vi "4461 Replace AO Ch.vi"(8 "error in (no error)":errorcluster, 10 "Lockin.DAQ (NEW)":refnum<class "Lockin.DAQ.lvclass">, 11 "Lockin.DAQ (OLD)":refnum<class "Lockin.DAQ.lvclass">) -> (0 "error out":errorcluster, 3 "Lockin.DAQ out":refnum<class "Lockin.DAQ.lvclass">)   [LabVIEW 2016, in "Lockin.DAQ.lvclass"]
uses:
  Lockin.DAQ.lvclass
  Lockin.DAQ.lvclass/Lockin.DAQ.ctl
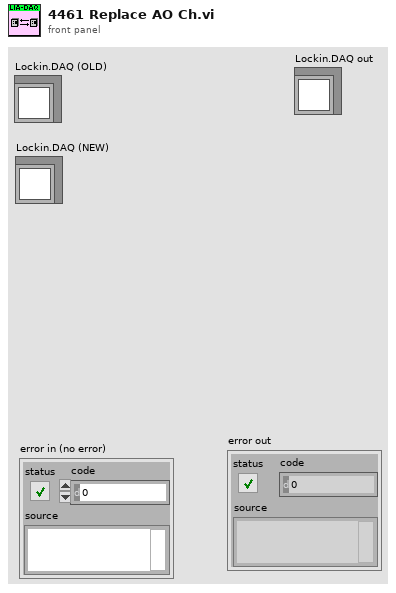
[diagram p1: front panel]
types:
  T1 = typedef "Lockin.DAQ.lvclass/AO-cluster.ctl" = cluster{"Ch":i32[], "Amp (V)":dbl[], "DC (V)":dbl[], "f (Hz)":dbl[], "Phase (°)":dbl[], "Function":T2[], "Sweep?":bool[]}
  T2 = typedef "Lockin.DAQ.lvclass/Function-enum.ctl" = enum16{"Sine", "Triangle", "Square", "Sawtooth"}
  T3 = typedef "Lockin.DAQ.lvclass/REF-cluster.ctl" = cluster{"Ch":i32[], " f (Hz)":dbl[], "Phase (°)":dbl[], "TC (s)":dbl[], "order":i32[]}
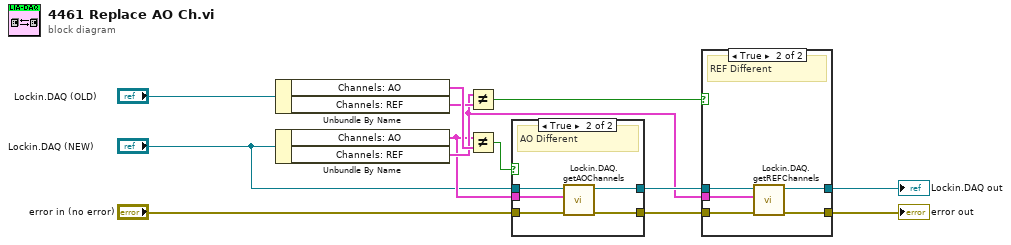
[diagram p0: block diagram]
diagram:
  n1 = Unbundle By Name("Lockin.DAQ (OLD)") -> ("Channels: AO"=w12:T1, "Channels: REF"=w11:T3)
  n2 = Unbundle By Name("Lockin.DAQ (NEW)") -> ("Channels: AO"=w2:T1, "Channels: REF"=w3:T3)
  n3 = Not Equal?(x=w3, y=w11) -> (x != y?=w9:bool)
  n4 = Not Equal?(x=w2, y=w12) -> (x != y?=w10:bool)
  n5 = case shown="True" w10 {
    tunnel: [w15 w19] -> w7
    tunnel: "Lockin.DAQ (NEW)" -> [w15 w20]
    tunnel: "error in (no error)" -> [w14 w18]
    tunnel: [w14 w17] -> w5
    tunnel: w2 -> [_ w16]
    frame False {
    }
    frame True {
      # "AO Different"
      n6 = call "Lockin.DAQ.getAOChannels.vi"("error in (no error)"=w18, "Channels: AO"=w16, "LockinDAQ"=w20) -> ("error out"=w17:errorcluster, "LockinDAQ out"=w19:refnum<class "Lockin.DAQ.lvclass">)  [unwired: 7 in]
    }
  }
  n7 = case shown="True" w9 {
    tunnel: [w22 w26] -> w8
    tunnel: w7 -> [w22 w27]
    tunnel: w5 -> [w21 w25]
    tunnel: [w21 w24] -> w4
    tunnel: w3 -> [_ w23]
    frame False {
    }
    frame True {
      # "REF Different"
      n8 = call "Lockin.DAQ.getREFChannels.vi"("error in (no error)"=w25, "Channels: REF"=w23, "LockinDAQ"=w27) -> ("error out"=w24:errorcluster, "LockinDAQ out"=w26:refnum<class "Lockin.DAQ.lvclass">)  [unwired: 7 in]
    }
  }
  "Lockin.DAQ out" <- w8
  "error out" <- w4
